vi "5RobotsRole.vi"(6 "Position":dbl, 7 "firstCall":bool, 8 "error in (no error)":errorcluster, 10 "Game in":refnum<class "Game.lvclass">, 11 "5RobotsRole in":refnum<class "5RobotsRole.lvclass">) -> (0 "error out":errorcluster, 3 "5RobotsRole out":refnum<class "5RobotsRole.lvclass">, 5 "Robot out":refnum<class "Robot.lvclass">)   [LabVIEW 2020, in "5RobotsRole.lvclass"]
uses:
  5RobotsRole.lvclass
  C:/Users/pipew/OneDrive/Documentos/GitHub/SSL_AI/Role_class/Role.lvclass
  Robot_class/Robot.lvclass
  Game_class/Game.lvclass
  Role_class/Role.lvclass/Role.ctl
  ShootTactic_class/States.ctl
  Role_class/Read Tacticbook.vi
  Role_class/Write Tacticbook.vi
  Role_class/Write tactic_index.vi
  Role_class/Read RobotRef.vi
  Tacticbook_class/Tacticbook.lvclass
  5RobotsTactic_class/5RobotsTactic.lvclass
  ShootTactic_class/ShootTactic.lvclass
panel:
  out "Game out":refnum<class "Game.lvclass">
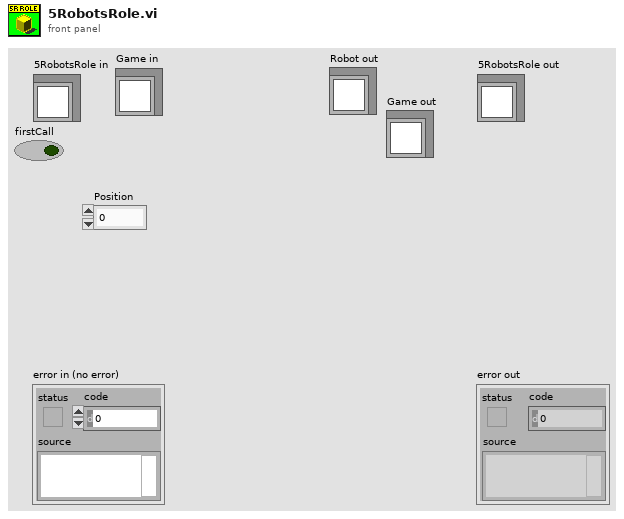
[diagram p1: front panel]
types:
  T1 = typedef "ShootTactic.lvclass/States.ctl" = enum16{"BallInGoalieArea", "Exit", "KickToGoal", "StealBall"}
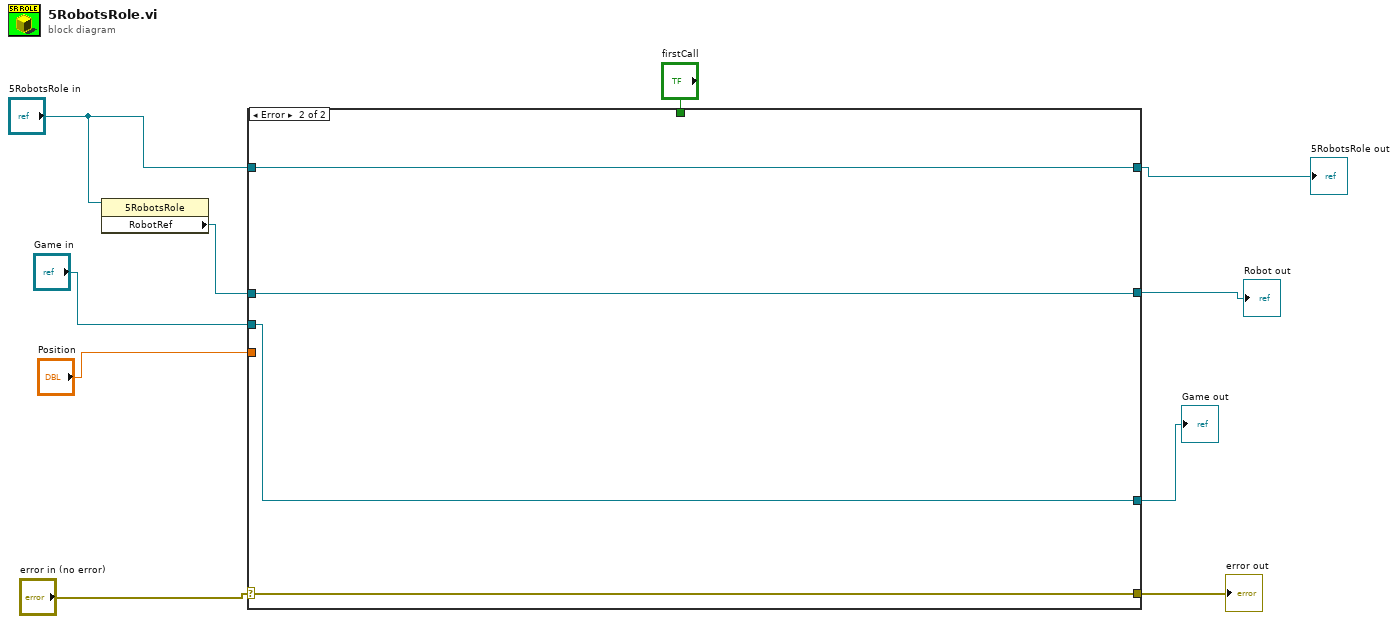
[diagram p0: block diagram]
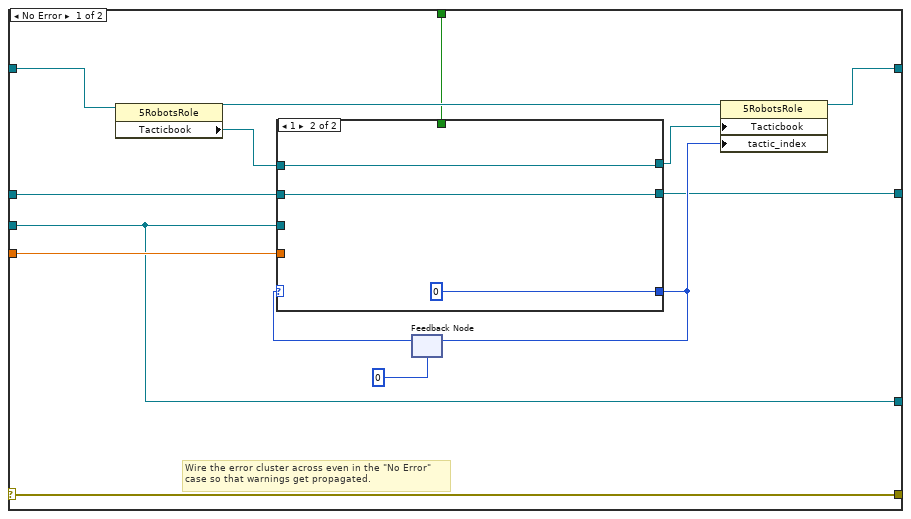
[diagram p2: hidden frame]
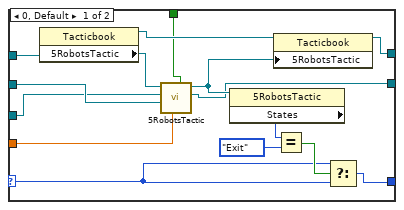
[diagram p3: hidden frame]
diagram:
  n1 = property class="5RobotsRole"(reference="5RobotsRole in") -> ("RobotRef"=w5:refnum<class "Robot.lvclass">)  [unwired: 1 in, 2 out]
  n2 = case shown="Error" "error in (no error)" {
    selector: "error in (no error)" -> [w24 w46]
    tunnel: [w24 w46] -> w8
    tunnel: [w17 w45] -> w10
    tunnel: "5RobotsRole in" -> [w16 w45]
    tunnel: "firstCall" -> [w15 _]
    tunnel: w5 -> [w14 w44]
    tunnel: "Game in" -> [w12 w43]
    tunnel: "Position" -> [w13 _]
    tunnel: [w12 w43] -> w2
    tunnel: [w11 w44] -> w1
    frame No Error {
      # "Wire the error cluster across even in the \"No Error\"\ncase so that warnings get propagated."
      n3 = property class="5RobotsRole"(reference=w16) -> (reference out=w23:refnum<class "5RobotsRole.lvclass">, "Tacticbook"=w20:refnum<class "Tacticbook.lvclass">)  [unwired: 1 in, 1 out]
      n4 = feedback #1(0) -> (w21:i32)
      n5 = case shown="1" w21 {
        selector: w21 -> [w32 _]
        tunnel: [w36 0] -> w19
        tunnel: w20 -> [w39 w41]
        tunnel: [w34 w41] -> w18
        tunnel: w15 -> [w26 _]
        tunnel: w14 -> [w29 w40]
        tunnel: w12 -> [w28 _]
        tunnel: w13 -> [w27 _]
        tunnel: [w25 w40] -> w11
        frame 0, Default {
          n6 = property class="Tacticbook"(reference=w39) -> (reference out=w35:refnum<class "Tacticbook.lvclass">, "5RobotsTactic"=w31:refnum<class "5RobotsTactic.lvclass">)  [unwired: 1 in, 1 out]
          n7 = call "5RobotsTactic.vi"("firstCall"=w26, "Position"=w27, "Robot In"=w29, "Game in"=w28, "5RobotsTactic in"=w31) -> ("Robot out"=w25:refnum<class "Robot.lvclass">, "5RobotsTactic out"=w30:refnum<class "5RobotsTactic.lvclass">)  [unwired: 4 in, 1 out]
          n8 = property class="5RobotsTactic"(reference=w30) -> ("States"=w38:enum16{"Position", "Exit"})  [unwired: 1 in, 2 out]
          n9 = property class="Tacticbook"(reference=w35, "5RobotsTactic"=w30) -> (reference out=w34:refnum<class "Tacticbook.lvclass">)  [unwired: 1 in, 1 out]
          n10 = Equal?(x=w38, y=States."Exit") -> (x = y?=w37:bool)
          n11 = Select(t=w32, s=w37, f=w32) -> (s? t:f=w36:i32)
        }
        frame 1 {
        }
      }
      n12 = feedback-in #1(w19) -> ()
      n13 = property class="5RobotsRole"(reference=w23, "Tacticbook"=w18, "tactic_index"=w19) -> (reference out=w17:refnum<class "5RobotsRole.lvclass">)  [unwired: 1 in, 1 out]
    }
    frame Error {
    }
  }
  "error out" <- w8
  "5RobotsRole out" <- w10
  "Robot out" <- w1
  "Game out" <- w2
